vi "One Cycle.vi"(1 "In":bool) -> (0 "Out":bool)   [LabVIEW 2015]
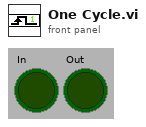
[diagram p1: front panel]
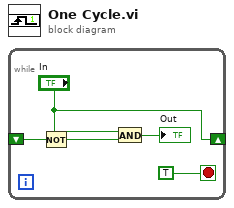
[diagram p0: block diagram]
diagram:
  n1 = while {
    shift-right: ["In"] -> _
    shift-left: _ -> [w2]
    stop <- TRUE stop-if-true
    n2 = Not(x=w2) -> (.not. x?=w4:bool)
    n3 = And(x="In", y=w4) -> (x .and. y?=→"Out":bool)
  }
